vi "PRIME Telescope Get Status.vi"(8 "error in (no error)":errorcluster, 11 "connection ID":refnum<k5>) -> (0 "error out":errorcluster, 1 "msg timestamp":timestamp, 2 "Raw Response":string, 3 "Telescope Status":T1, 4 "Cmd":string="A 001 004 009 018 020 017\r")   [LabVIEW 2024, in "PRIME Telescope.lvclass"]
uses:
  PRIME Telescope.lvclass
  Telescope cluster Status.ctl
  typedefs/CC cluster RA and DEC.ctl
  Telescope enum Status.ctl
  Telescope.lvclass
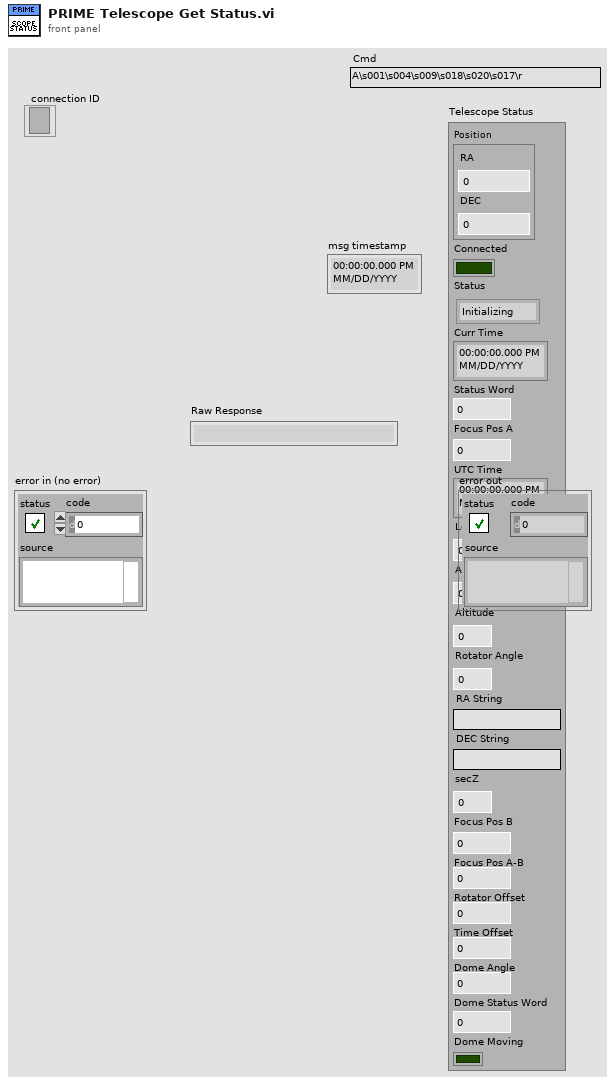
[diagram p1: front panel]
types:
  T1 = typedef "Telescope.lvclass/Telescope cluster Status.ctl" = cluster{"Position":T2, "Connected":bool, "Status":T3, "Curr Time":timestamp, "Status Word":u32, "Focus Pos A":dbl, "UTC Time":timestamp, "Local Sidreal Time":dbl, "Azimuth":dbl, "Altitude":dbl, "Rotator Angle":dbl, "RA String":string, "DEC String":string, "secZ":dbl, "Focus Pos B":dbl, "Focus Pos A-B":dbl, "Rotator Offset":dbl, "Time Offset":dbl, "Dome Angle":dbl, "Dome Status Word":u32, "Dome Moving":bool}
  T2 = typedef "CC cluster RA and DEC.ctl" = cluster{"RA":dbl, "DEC":dbl}
  T3 = typedef "Telescope.lvclass/Telescope enum Status.ctl" = enum16{"Initializing", "Ready", "Moving", "Focusing", "Error"}
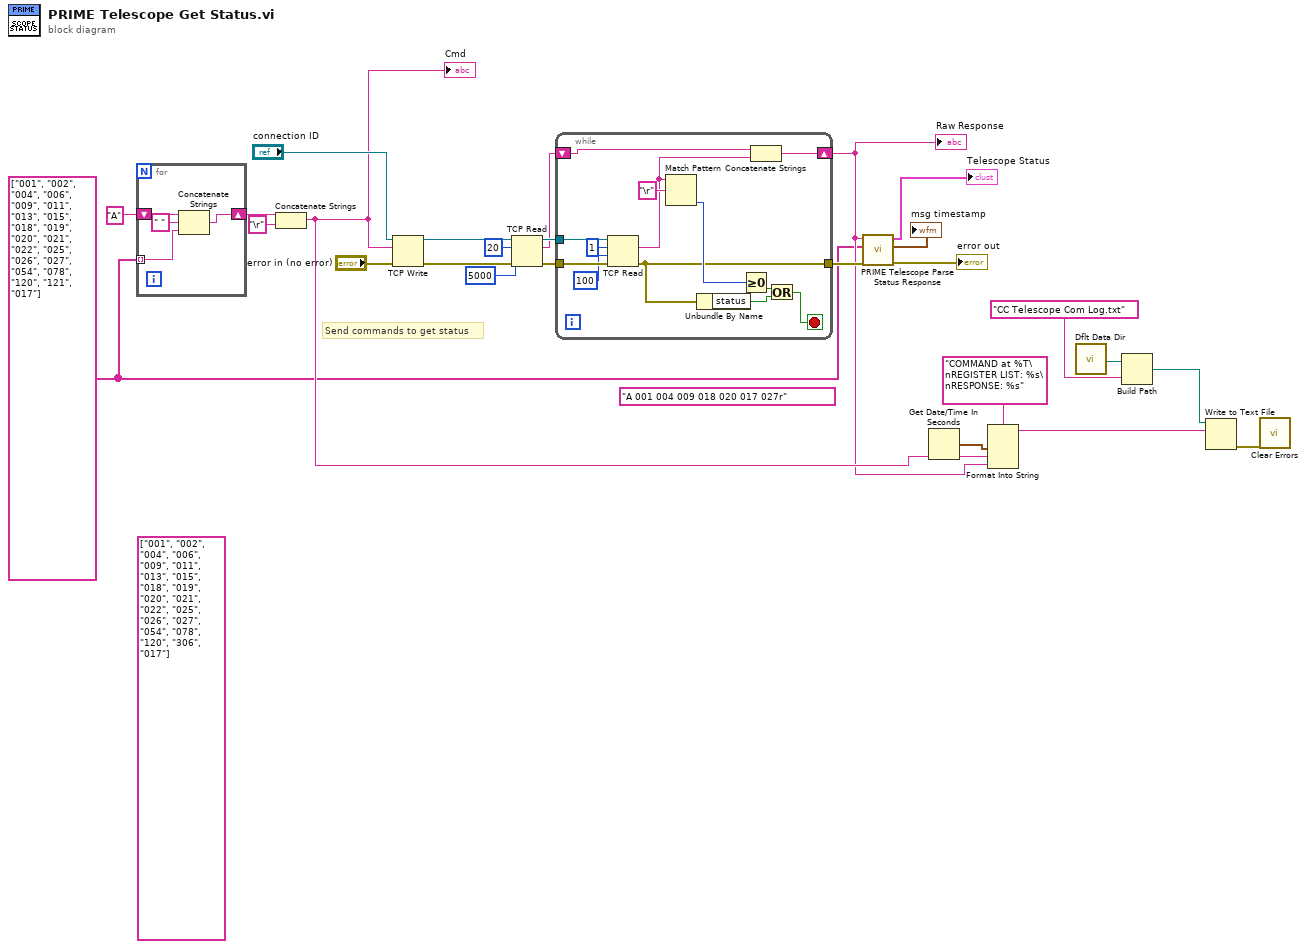
[diagram p0: block diagram]
diagram:
  (unwired) string[] ["001", "002", "004", "006", "009", "011", "013", "015", "018", "019", "020", "021", "022", "025", "026", "027", "054", "078", "120", "306", "017"]
  w1 = string[] ["001", "002", "004", "006", "009", "011", "013", "015", "018", "019", "020", "021", "022", "025", "026", "027", "054", "078", "120", "121", "017"]
  (unwired) "A 001 004 009 018 020 017 027r"
  # "Send commands to get status"
  n1 = for {
    tunnel: w1 -> [w28] mode=indexing
    shift-right: [w27] -> w12
    shift-left: "A" -> [w30]
    n2 = Concatenate Strings(w30, " " ("string"), w28) -> (w27:string)
  }
  n3 = Concatenate Strings(w12, "\r" ("string")) -> (w8:string)
  "Cmd" <- w8
  n4 = TCP Write(connection ID="connection ID", data in=w8, error in (no error)="error in (no error)") -> (connection ID out=w24:refnum<k5>, error out=w23:errorcluster)  [unwired: 1 in, 1 out]
  n5 = TCP Read(connection ID=w24, bytes to read=20, error in (no error)=w23, 9:5000 ("timeout ms (25000)")) -> (connection ID out=w16:refnum<k5>, data out=w15:string, error out=w17:errorcluster)  [unwired: 1 in]
  n6 = while {
    tunnel: w17 -> [w42]
    tunnel: w16 -> [w43]
    shift-right: [w32] -> w7
    shift-left: w15 -> [w34]
    tunnel: [w31] -> w14
    stop <- w35 stop-if-true
    n7 = TCP Read(connection ID=w43, bytes to read=1, error in (no error)=w42, 9:100 ("timeout ms (25000)")) -> (data out=w33:string, error out=w31:errorcluster)  [unwired: 1 in, 1 out]
    n8 = Match Pattern(string=w33, regular expression="\r") -> (offset past match=w38:i32)  [unwired: 1 in, 3 out]
    n9 = Unbundle By Name(w31) -> ("status"=w36:bool)
    n10 = Greater Or Equal To 0?(x=w38) -> (x >= 0?=w37:bool)
    n11 = Concatenate Strings(w34, w33) -> (w32:string)
    n12 = Or(x=w37, y=w36) -> (x .or. y?=w35:bool)
  }
  "Raw Response" <- w7
  n13 = call "PRIME Telescope Parse Status Response.vi"("error in"=w14, "Reg List"=w1, "input string"=w7) -> ("error out"=→"error out":errorcluster, "msg timestamp"=→"msg timestamp":timestamp, "Telescope Status"=→"Telescope Status":T1)  [unwired: 6 in]
  n14 = Get Date/Time In Seconds() -> (seconds since 1Jan1904=w9:timestamp)
  n15 = Format Into String(format string="COMMAND at %T\nREGISTER LIST: %s\nRESPONSE: %s", w9, w8, w7) -> (resulting string=w6:string)  [unwired: 2 in, 1 out]
  n16 = call <vilib>:"Dflt Data Dir.vi"() -> ("App:Default Data Directory"=w5:path)
  n17 = Build Path(base path=w5, name or relative path="CC Telescope Com Log.txt") -> (appended path=w3:path)
  n18 = Write to Text File(file (use dialog)=w3, text=w6) -> (error out=w2:errorcluster)  [unwired: 2 in, 2 out]
  n19 = call <vilib>:"Clear Errors.vi"("error in (no error)"=w2) -> ()  [unwired: 5 in, 2 out]
